vi "Test To Report Entry.vi"(8 "error in (no error)":errorcluster, 10 "Test Node":T1) -> (0 "error out":errorcluster, 2 "String":string)   [LabVIEW 2020, in "Caraya.lvlib" / "Test Report.Default.lvclass"]
uses:
  Test Report.Default.lvclass
  Test Result/Test Node (Extended).ctl
  Test Result/Test Registration Data.ctl
  Test Report/Test Report.lvclass
  Test Report.Event/Test Report.Event.lvclass
  Test Result/Test Result.lvclass
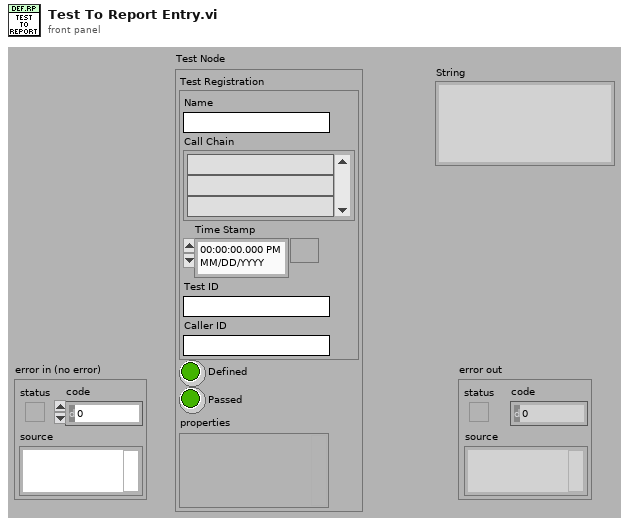
[diagram p1: front panel]
types:
  T1 = typedef "Caraya.lvlib/Test Result.lvclass/Test Node (Extended).ctl" = cluster{"Test Registration":T2, "Defined":bool, "Passed":bool, "properties":variant}
  T2 = typedef "Caraya.lvlib/Test Result.lvclass/Test Registration Data.ctl" = cluster{"Name":string, "Call Chain":string[], "Time Stamp":timestamp, "Test ID":string, "Caller ID":string}
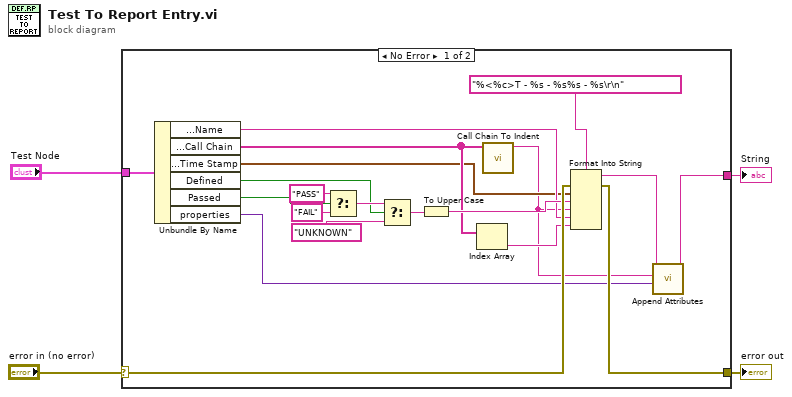
[diagram p0: block diagram]
diagram:
  n1 = case shown="No Error" "error in (no error)" {
    selector: "error in (no error)" -> [w22 w25]
    tunnel: [w21 w25] -> w3
    tunnel: "Test Node" -> [w24 _]
    tunnel: [w6 _] -> w1
    frame No Error {
      n2 = Unbundle By Name(w24) -> ("Test Registration.Name"=w18:string, "Test Registration.Call Chain"=w19:string[], "Test Registration.Time Stamp"=w16:timestamp, "Defined"=w11:bool, "Passed"=w13:bool, "properties"=w8:variant)
      n3 = Select(t="PASS" ("format string"), s=w13, f="FAIL" ("format string")) -> (s? t:f=w15:string)
      n4 = Select(t=w15, s=w11, f="UNKNOWN" ("format string")) -> (s? t:f=w9:string)
      n5 = To Upper Case(1:w9) -> (0:w20:string)
      n6 = Index Array(array=w19) -> (element=w17:string)  [unwired: 1 in]
      n7 = call "Call Chain To Indent.vi"("Call Chain"=w19) -> ("Indent"=w5:string)  [unwired: 10 in]
      n8 = Format Into String(format string="%<%c>T - %s - %s%s - %s\r\n", error in=w22, w16, w20, w5, w18, w17) -> (resulting string=w7:string, error out=w21:errorcluster)  [unwired: 1 in]
      n9 = call "Append Attributes.vi"("attributes"=w8, "Indent"=w5, "String in"=w7) -> ("String out"=w6:string)  [unwired: 7 in, 1 out]
    }
    frame Error {
    }
  }
  "error out" <- w3
  "String" <- w1
